vi "Final Circle Drawing.vi"(8 "picture":picture, 9 "Actual values":dbl[](array[numeric]), 10 "Horizontal summary":dbl, 11 "Vertical summary":dbl) -> (0 "ADC0":dbl, 1 "ADC2":dbl, 2 "ADC1":dbl, 3 "ADC3":dbl, 4 "ADC Chart":cluster{dbl, dbl, dbl, dbl}, 5 "Img result":picture)   [LabVIEW 2014]
panel:
  out "in - out":bool
  in  "color - out":u32(colorbox)=16711680
  in  "pen- out":T1={"Width"=3, "Style"=enum."Dash"}
  in  "color - in":u32(colorbox)=6618880
  in  "pen - in":T1={"Width"=4, "Style"=enum."Solid"}
  out "ADC0":dbl
  out "ADC2":dbl
  out "ADC1":dbl
  out "ADC3":dbl
  in  "pen - dot":T1={"Width"=6, "Style"=enum."Solid"}
  in  "color - dot":u32(colorbox)=16711835
  in  "radius":i16=150
  in  "point(x,y)":cluster{"x":i16, "y":i16}
  # "Actual values"
  # "Previous values"
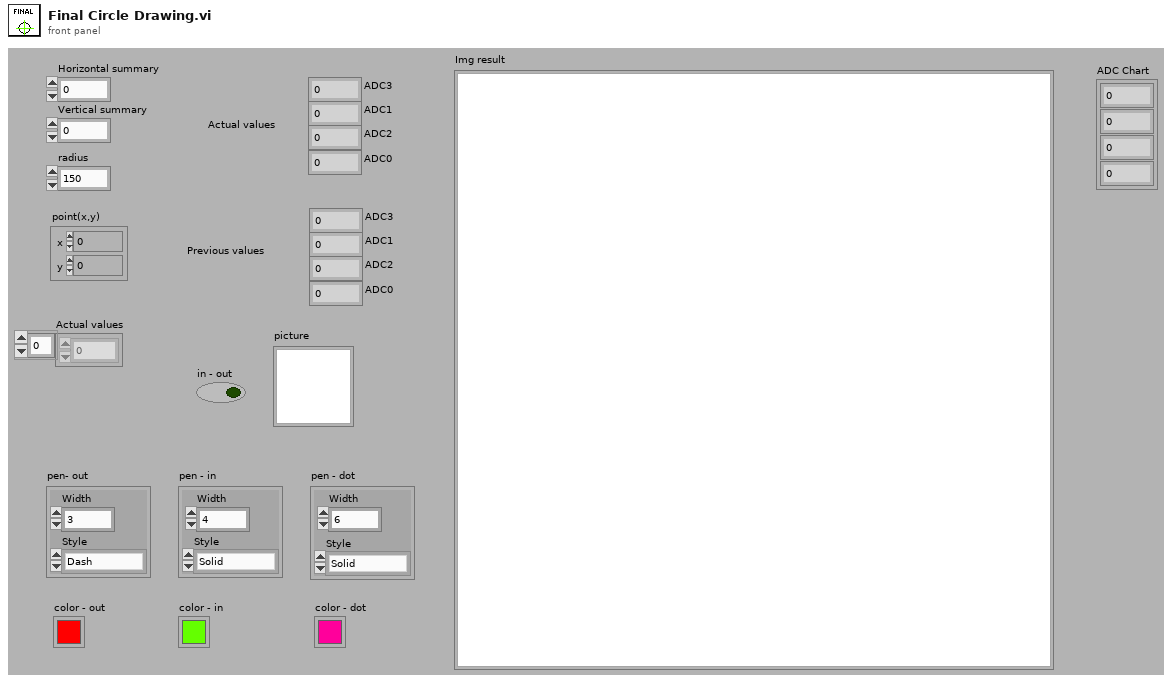
[diagram p1: front panel]
types:
  T1 = cluster{"Width":u16, "Style":enum32{"Solid", "Dash", "Dot", "DashDot", "DashDotDot"}}
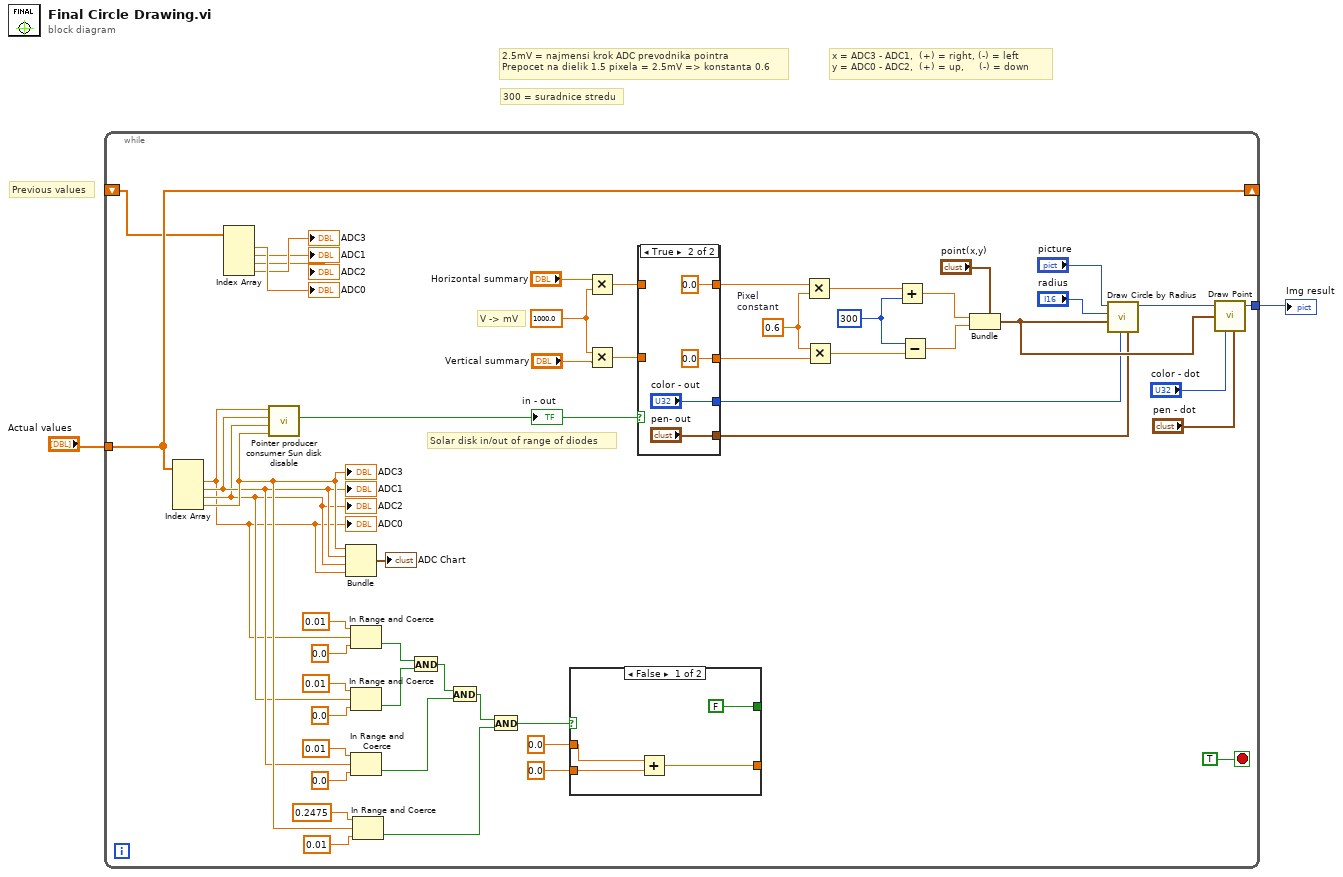
[diagram p0: block diagram]
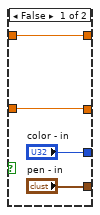
[diagram p2: hidden frame]
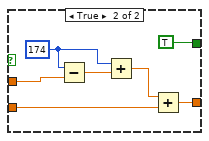
[diagram p3: hidden frame]
diagram:
  # "Previous values"
  # "x = ADC3 - ADC1,  (+) = right, (-) = left \ny = ADC0 - ADC2,  (+) = up,     (-) = down"
  # "300 = suradnice stredu"
  # "2.5mV = najmensi krok ADC prevodnika pointra\nPrepocet na dielik 1.5 pixela = 2.5mV => konstanta 0.6"
  n1 = while {
    tunnel: [w51] -> w2
    tunnel: "Actual values" -> [w14]
    shift-right: [w14] -> _
    shift-left: _ -> [w13]
    stop <- TRUE stop-if-true
    w37 = 1000.0 ("x")
    w54 = 0.6  # Pixel  constant
    w43 = 300
    # "V -> mV"
    # "Solar disk in/out of range of diodes"
    n2 = Index Array(array=w14) -> (element #1=w4:dbl, element #2=w6:dbl, element #3=w5:dbl, element #4=w7:dbl)  [unwired: 4 in]
    "ADC3" <- w7
    "ADC1" <- w6
    "ADC2" <- w5
    "ADC0" <- w4
    n3 = Index Array(array=w13) -> (element #1=→"ADC0":dbl, element #2=→"ADC1":dbl, element #3=→"ADC2":dbl, element #4=→"ADC3":dbl)  [unwired: 4 in]
    n4 = call "Pointer producer consumer Sun disk disable.vi"("ADC0"=w4, "ADC1"=w6, "ADC2"=w5, "ADC3"=w7) -> ("in - out"=w8:bool)  [unwired: 4 in]
    "in - out" <- w8
    n5 = Bundle(w7, w6, w5, w4) -> (→"ADC Chart":cluster{dbl, dbl, dbl, dbl})  [unwired: 1 in]
    n6 = In Range and Coerce(upper limit=0.01 ("x"), x=w4, lower limit=0.0 ("x")) -> (In Range?=w24:bool)  [unwired: 1 out]
    n7 = In Range and Coerce(upper limit=0.01 ("x"), x=w5, lower limit=0.0 ("x")) -> (In Range?=w23:bool)  [unwired: 1 out]
    n8 = In Range and Coerce(upper limit=0.01 ("x"), x=w6, lower limit=0.0 ("x")) -> (In Range?=w22:bool)  [unwired: 1 out]
    n9 = In Range and Coerce(upper limit=0.2475 ("x"), x=w7, lower limit=0.01 ("x")) -> (In Range?=w17:bool)  [unwired: 1 out]
    n10 = And(x=w24, y=w23) -> (x .and. y?=w21:bool)
    n11 = And(x=w21, y=w22) -> (x .and. y?=w18:bool)
    n12 = And(x=w18, y=w17) -> (x .and. y?=w16:bool)
    n13 = case shown="False" w16 {
      tunnel: [w67 w74] -> _
      tunnel: [FALSE TRUE] -> _
      tunnel: 0.0 ("Horizontal summary") -> [w65 w69]
      tunnel: 0.0 ("Horizontal summary") -> [w64 w68]
      frame False {
        n14 = Add(x=w65, y=w64) -> (x+y=w67:dbl)
      }
      frame True {
        w72 = 174
        n15 = Subtract(x=w72, y=w69) -> (x-y=w73:dbl)
        n16 = Add(x=w72, y=w73) -> (x+y=w71:dbl)
        n17 = Add(x=w71, y=w68) -> (x+y=w74:dbl)
      }
    }
    n18 = Multiply(x="Horizontal summary", y=w37) -> (x*y=w36:dbl)
    n19 = Multiply(x=w37, y="Vertical summary") -> (x*y=w35:dbl)
    n20 = case shown="True" w8 {
      tunnel: ["color - in" "color - out"] -> w38
      tunnel: ["pen - in" "pen- out"] -> w39
      tunnel: w36 -> [w57 _]
      tunnel: [w57 0.0 ("Horizontal summary")] -> w41
      tunnel: [w56 0.0 ("Vertical summary")] -> w40
      tunnel: w35 -> [w56 _]
      frame False {
      }
      frame True {
      }
    }
    n21 = Multiply(x=w41, y=w54) -> (x*y=w44:dbl)
    n22 = Multiply(x=w54, y=w40) -> (x*y=w46:dbl)
    n23 = Add(x=w44, y=w43) -> (x+y=w42:dbl)
    n24 = Subtract(x=w43, y=w46) -> (x-y=w45:dbl)
    n25 = Bundle(cluster="point(x,y)", "x"=w42, "y"=w45) -> (w47:cluster{"x":i16, "y":i16})
    n26 = call <vilib>:"Draw Circle by Radius.vi"("pen"=w39, "color(black)"=w38, "pixel center"=w47, "radius"="radius", "picture"="picture") -> ("new picture"=w52:picture)  [unwired: 6 in]
    n27 = call <vilib>:"Draw Point.vi"("picture"=w52, "point(x,y)"=w47, "color(black)"="color - dot", "pen"="pen - dot") -> ("new picture"=w51:picture)  [unwired: 5 in]
  }
  "Img result" <- w2
